vi "system.vi"() -> ()   [LabVIEW 2011]
uses:
  <vilib>/httpClient/POSTBuffer.vi
  <vilib>/httpClient/LabVIEWHTTPClient.lvlib
panel:
  in  "odswiez":bool
  in  "usunZdjecia":bool
  in  "usunZdjecie":bool
  in  "restartSystemu":bool
  in  "stopSystemu":bool
  in  "startSystemu":bool
  out "statusSystemu":bool
  in  "usunAlarmy":bool
  in  "usunAlarm":bool
  in  "alarmyRing":u16(ring) items=["2015-02-03 14:53:43"]
  out "picturesDir":string
  out "konfiguracja":string[][](array[string])
  out "alarmyString":string
  out "zdjecie":picture
  in  "zdjeciaRing":u16(ring) items=["2015-02-03 14:53:43.556413.jpg", "2015-02-03 14:53:45.230714.jpg", "2015-02-03 14:53:45.560907.jpg", "2015-02-03 14:53:45.893951.jpg", "2015-02-03 14:53:46.227903.jpg", "2015-02-03 14:53:46.565637.jpg", "2015-02-03 14:53:46.897487.jpg", "2015-02-03 14:53:47.231445.jpg", "2015-02-03 14:53:47.565422.jpg", "2015-02-03 14:53:47.899491.jpg", "2015-02-03 14:53:48.233446.jpg", "2015-02-03 14:53:48.567392.jpg", "2015-02-03 14:53:48.901593.jpg", "2015-02-03 14:53:49.235569.jpg", "2015-02-03 14:53:49.569530.jpg", "2015-02-03 14:53:49.903480.jpg", "2015-02-03 14:53:50.256797.jpg", "2015-02-03 14:53:50.571229.jpg", "2015-02-03 14:53:50.905749.jpg", "2015-02-03 14:53:51.239702.jpg", "2015-02-03 14:53:51.573789.jpg", "2015-02-03 14:53:51.907839.jpg"]
  in  "Zapisz":bool
  in  "edytujKonfiguracje":u16(ring) items=["logAlarms", "sendEmail", "senderEmail", "receiverEmail", "emailSubject", "picturesPerSecond"]
  in  "edytujKonfiguracje":string
  in  "Polacz":bool
  in  "Hasło:":string
  in  "Login:":string
  in  "IP:":string
  # "Przeglądaj zdjęcia:"
  # "Status systemu:"
  # "Wykryte alarmy:"
  # "Konfiguracja:"
  # "Zarządzaj alarmami:"
  # "Zarządzaj konfiguracją:"
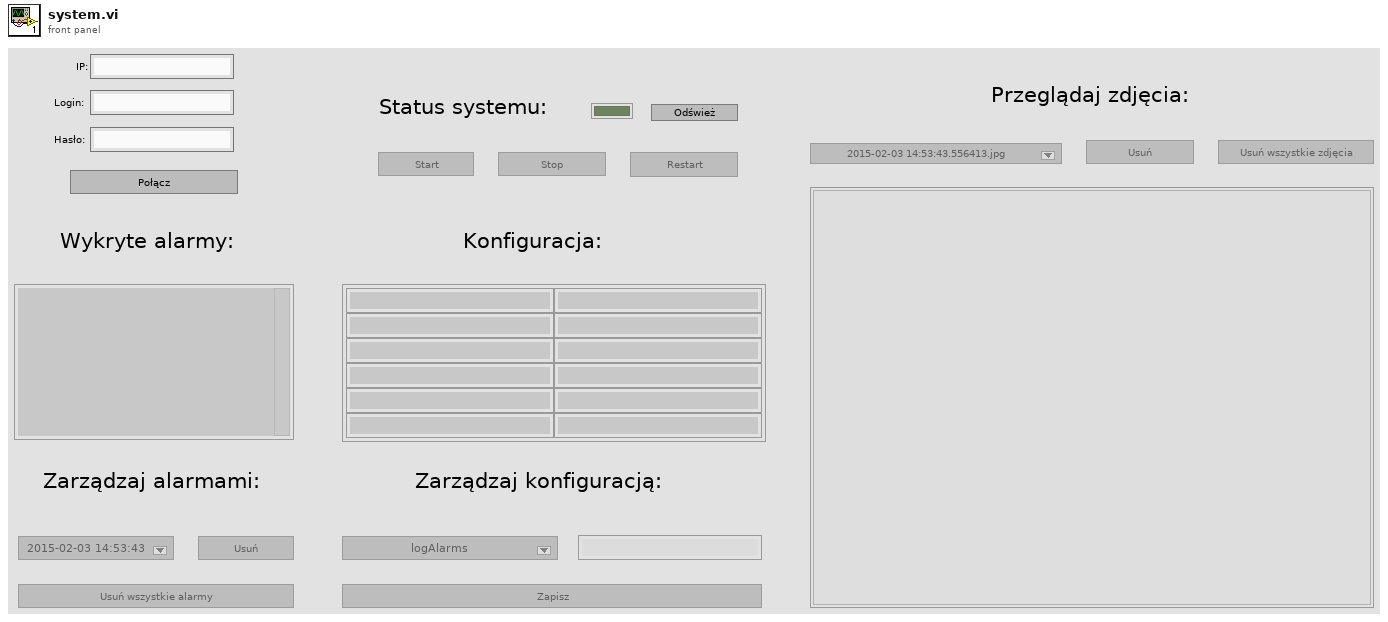
[diagram p1: front panel]
types:
  T1 = enum8{"Enabled", "Disabled", "Disabled and Grayed Out"}
  T2 = enum16{"open", "open or create", "create or replace", "create", "open (read only)"}
  T3 = typedef "LVBoundsTypeDef.ctl" = cluster{"Width":u32, "Height":u32}
  T4 = typedef "imagedata.ctl" = cluster{"image type":i32, "image depth":i32, "image":u8[], "mask":u8[], "colors":u32[], "Rectangle":cluster{"left":i16, "top":i16, "right":i16, "bottom":i16}}
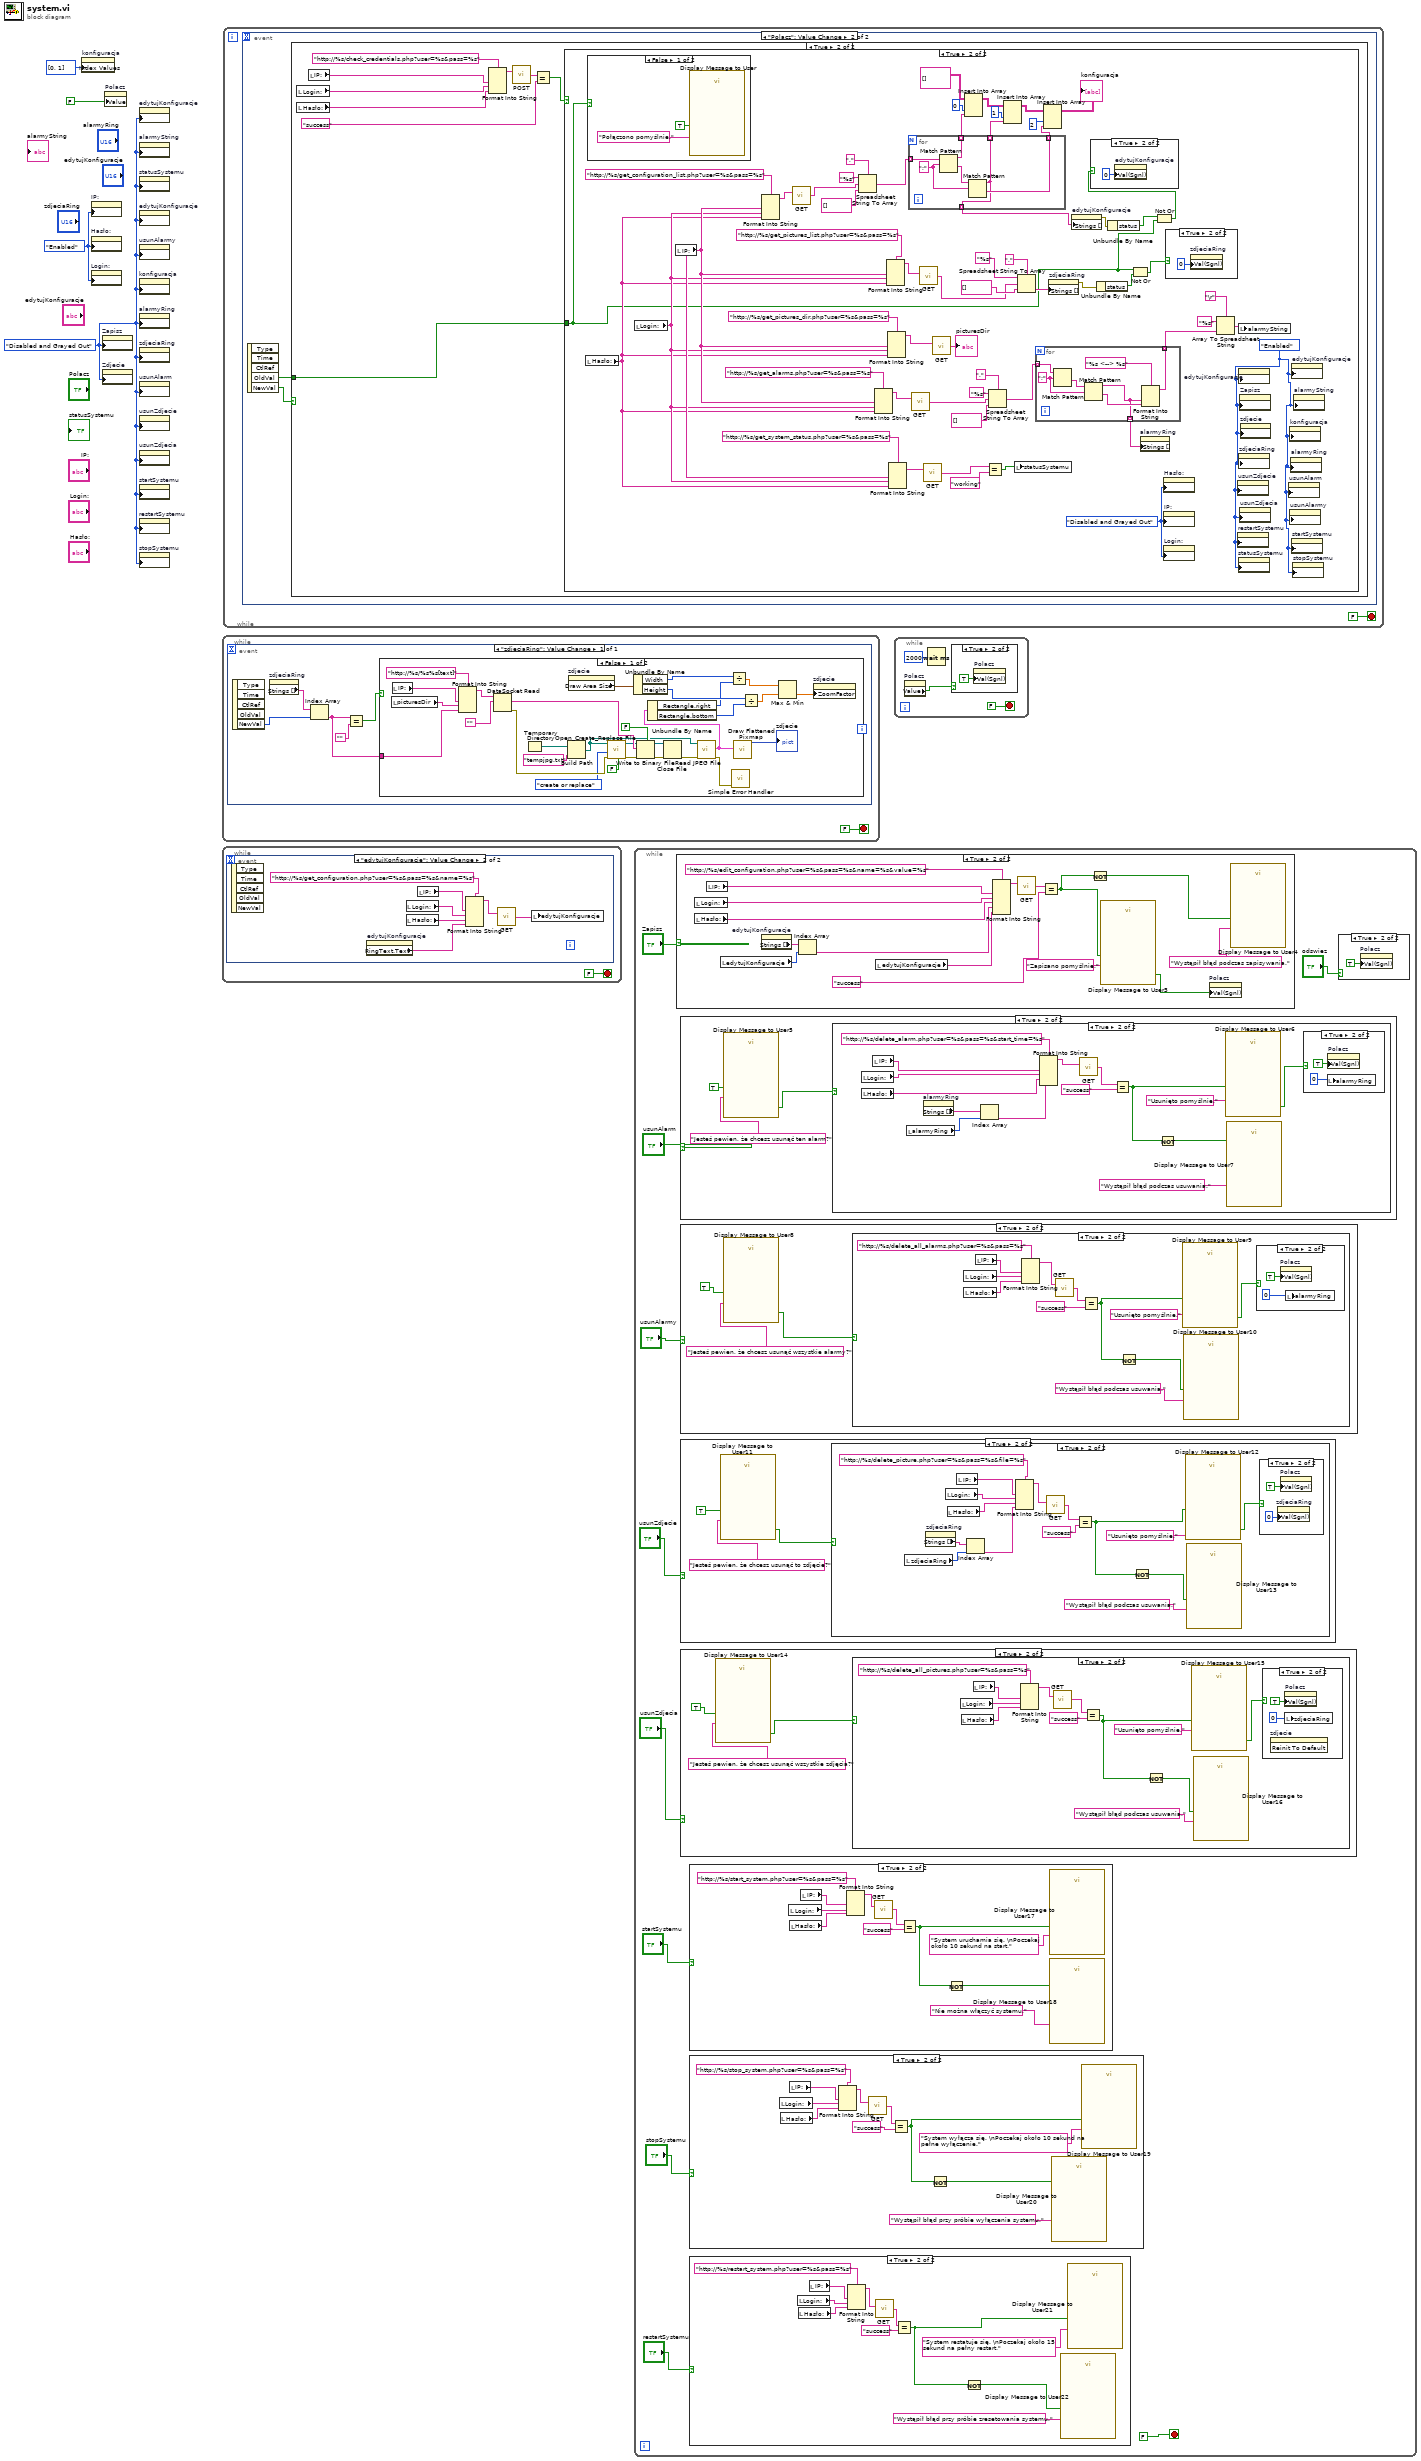
[diagram p0: block diagram]
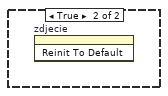
[diagram p3: hidden frame]
diagram:
  w2 = T1."Disabled and Grayed Out" ("Disabled")
  w4 = T1."Enabled" ("Disabled")
  n1 = property on="konfiguracja" class="Arr (strict)"("Index Values"=u32[] [0, 1]) -> ()  [unwired: 2 in, 2 out]
  n2 = property on="IP:" class="Str"("DisabledEnum"=w4) -> ()  [unwired: 2 in, 2 out]
  n3 = property on="Hasło:" class="Str"("DisabledEnum"=w4) -> ()  [unwired: 2 in, 2 out]
  n4 = property on="Login:" class="Str"("DisabledEnum"=w4) -> ()  [unwired: 2 in, 2 out]
  n5 = property on="Zapisz" class="Bool"("DisabledEnum"=w2) -> ()  [unwired: 2 in, 2 out]
  n6 = property on="Zdjecie" class="Pict"("DisabledEnum"=w2) -> ()  [unwired: 2 in, 2 out]
  n7 = property on="Polacz" class="Bool (strict)"("Value"=FALSE ("Polacz")) -> ()  [unwired: 2 in, 2 out]
  n8 = property on="edytujKonfiguracje" class="Str"("DisabledEnum"=w2) -> ()  [unwired: 2 in, 2 out]
  n9 = property on="alarmyString" class="Str"("DisabledEnum"=w2) -> ()  [unwired: 2 in, 2 out]
  n10 = property on="statusSystemu" class="Bool (strict)"("DisabledEnum"=w2) -> ()  [unwired: 2 in, 2 out]
  n11 = property on="edytujKonfiguracje" class="Ring (strict)"("DisabledEnum"=w2) -> ()  [unwired: 2 in, 2 out]
  n12 = property on="usunAlarmy" class="Bool"("DisabledEnum"=w2) -> ()  [unwired: 2 in, 2 out]
  n13 = property on="konfiguracja" class="Arr (strict)"("DisabledEnum"=w2) -> ()  [unwired: 2 in, 2 out]
  n14 = property on="alarmyRing" class="Ring (strict)"("DisabledEnum"=w2) -> ()  [unwired: 2 in, 2 out]
  n15 = property on="zdjeciaRing" class="Ring (strict)"("DisabledEnum"=w2) -> ()  [unwired: 2 in, 2 out]
  n16 = property on="usunAlarm" class="Bool"("DisabledEnum"=w2) -> ()  [unwired: 2 in, 2 out]
  n17 = property on="usunZdjecie" class="Bool"("DisabledEnum"=w2) -> ()  [unwired: 2 in, 2 out]
  n18 = property on="usunZdjecia" class="Bool"("DisabledEnum"=w2) -> ()  [unwired: 2 in, 2 out]
  n19 = property on="startSystemu" class="Bool"("DisabledEnum"=w2) -> ()  [unwired: 2 in, 2 out]
  n20 = property on="restartSystemu" class="Bool"("DisabledEnum"=w2) -> ()  [unwired: 2 in, 2 out]
  n21 = property on="stopSystemu" class="Bool"("DisabledEnum"=w2) -> ()  [unwired: 2 in, 2 out]
  n22 = while {
    stop <- FALSE stop-if-true
    n23 = event shown="[0] \"zdjeciaRing\": Value Change" {
      selector: _ -> [_]
      dyn-events: _ -> [_]
      timeout: _ -> [_]
      event "zdjeciaRing": Value Change {
        n24 = event-data() -> ("NewVal"=w9:u16)  [unwired: 1 in, 4 out]
        n25 = property on="zdjeciaRing" class="Ring (strict)"() -> ("Strings []"=w10:string[])  [unwired: 2 in, 2 out]
        n26 = Index Array(array=w10, index=w9) -> (element=w7:string)
        n27 = Equal?(x=w7, y="") -> (x = y?=w6:bool)
        n28 = case shown="False" w6 {
          tunnel: w7 -> [w11 _]
          frame False {
            n29 = local read "picturesDir"() -> (w14:string)
            n30 = local read "IP:"() -> (w15:string)
            n31 = Format Into String(format string="http://%s/%s%s[text]", w15, w14, w11) -> (resulting string=w12:string)  [unwired: 2 in, 1 out]
            n32 = DataSocket Read(10:"", 11:w12) -> (0:w37:errorcluster, 2:w28:string)  [unwired: 3 in, 5 out]
            n33 = Temporary Directory() -> (w25:path)
            n34 = Build Path(base path=w25, name or relative path="tempjpg.txt") -> (appended path=w36:path)
            n35 = property on="zdjecie" class="Pict"() -> ("Draw Area Size"=w23:T3)  [unwired: 2 in, 2 out]
            n36 = call <vilib>:"Open_Create_Replace File.vi"("advisory dialog? (display:T)"=FALSE, "error in (no error)"=w37, "function (open:0)"=T2."create or replace", "file path"=w36) -> ("error out"=w29:errorcluster, "refnum"=w27:refnum<file>)  [unwired: 3 in, 3 out]
            n37 = Unbundle By Name(w23) -> ("Width"=w22:u32, "Height"=w21:u32)
            n38 = Write to Binary File(file (use dialog)=w27, data=w28, error in=w29, 5:FALSE ("prepend array or string size? (T)")) -> (refnum out=w31:refnum<file>, error out=w32:errorcluster)  [unwired: 3 out]
            n39 = Close File(refnum=w31, error in=w32) -> (error out=w33:errorcluster)  [unwired: 1 out]
            n40 = call <vilib>:"Read JPEG File.vi"("error in (no error)"=w33, "path to JPEG file"=w36) -> ("error out"=w30:errorcluster, "image data"=w40:T4)  [unwired: 8 out]
            n41 = Unbundle By Name(w40) -> ("Rectangle.right"=w19:i16, "Rectangle.bottom"=w20:i16)
            n42 = Divide(x=w22, y=w19) -> (x/y=w18:dbl)
            n43 = call <vilib>:"Simple Error Handler.vi"("error in (no error)"=w30) -> ()  [unwired: 1 in, 8 out]
            n44 = call <vilib>:"Draw Flattened Pixmap.vi"("image data"=w40) -> ("new picture"=→"zdjecie":picture)  [unwired: 3 in, 5 out]
            n45 = Divide(x=w21, y=w20) -> (x/y=w17:dbl)
            n46 = Max & Min(x=w18, y=w17) -> (min(x,y)=w16:dbl)  [unwired: 1 out]
            n47 = property on="zdjecie" class="Pict"("ZoomFactor"=w16) -> ()  [unwired: 2 in, 2 out]
          }
          frame True {
            n48 = invoke on="zdjecie" class="Pict" method="Reinit To Default"() -> ()  [unwired: 3 in, 3 out]
          }
        }
      }
    }
  }
  n49 = while {
    stop <- FALSE stop-if-true
    n50 = event shown="[1] \"edytujKonfiguracje\": Value Change" {
      selector: _ -> [_ _]
      dyn-events: _ -> [_ _]
      timeout: _ -> [_ _]
      event Timeout {
        n51 = event-data() -> ()  [unwired: 1 in, 2 out]
      }
      event "edytujKonfiguracje": Value Change {
        n52 = event-data() -> ()  [unwired: 1 in, 5 out]
        n53 = property on="edytujKonfiguracje" class="Ring (strict)"() -> ("RingText.Text"=w47:string)  [unwired: 2 in, 2 out]
        n54 = local read "Login:"() -> (w45:string)
        n55 = local read "Hasło:"() -> (w44:string)
        n56 = local read "IP:"() -> (w46:string)
        n57 = Format Into String(format string="http://%s/get_configuration.php?user=%s&pass=%s&name=%s" ("http URL"), w46, w45, w44, w47) -> (resulting string=w43:string)  [unwired: 2 in, 1 out]
        n58 = call <vilib>:"GET.vi"("url"=w43) -> ("body"=w42:string)  [unwired: 11 in, 3 out]
        n59 = local write "edytujKonfiguracje"(w42) -> ()
      }
    }
  }
  n60 = while {
    stop <- FALSE stop-if-true
    n61 = event shown="[1] \"Polacz\": Value Change" {
      selector: _ -> [_ _]
      dyn-events: _ -> [_ _]
      timeout: _ -> [_ _]
      event Timeout {
        n62 = event-data() -> ()  [unwired: 1 in, 2 out]
      }
      event "Polacz": Value Change {
        n63 = event-data() -> ("OldVal"=w50:bool, "NewVal"=w51:bool)  [unwired: 1 in, 3 out]
        n64 = case shown="True" w51 {
          tunnel: w50 -> [_ w54]
          frame False {
            w52 = T1."Disabled and Grayed Out" ("Disabled")
            w53 = T1."Enabled" ("Disabled")
            n65 = property on="Hasło:" class="Str"("DisabledEnum"=w53) -> ()  [unwired: 2 in, 2 out]
            n66 = property on="Login:" class="Str"("DisabledEnum"=w53) -> ()  [unwired: 2 in, 2 out]
            n67 = property on="IP:" class="Str"("DisabledEnum"=w53) -> ()  [unwired: 2 in, 2 out]
            n68 = property on="stopSystemu" class="Bool"("DisabledEnum"=w52) -> ()  [unwired: 2 in, 2 out]
            n69 = property on="restartSystemu" class="Bool"("DisabledEnum"=w52) -> ()  [unwired: 2 in, 2 out]
            n70 = property on="statusSystemu" class="Bool (strict)"("DisabledEnum"=w52) -> ()  [unwired: 2 in, 2 out]
            n71 = property on="alarmyRing" class="Ring (strict)"("DisabledEnum"=w52) -> ()  [unwired: 2 in, 2 out]
            n72 = property on="startSystemu" class="Bool"("DisabledEnum"=w52) -> ()  [unwired: 2 in, 2 out]
            n73 = property on="zdjecie" class="Pict"("DisabledEnum"=w52) -> ()  [unwired: 2 in, 2 out]
            n74 = property on="konfiguracja" class="Arr (strict)"("DisabledEnum"=w52) -> ()  [unwired: 2 in, 2 out]
            n75 = property on="edytujKonfiguracje" class="Str"("DisabledEnum"=w52) -> ()  [unwired: 2 in, 2 out]
            n76 = property on="zdjeciaRing" class="Ring (strict)"("DisabledEnum"=w52) -> ()  [unwired: 2 in, 2 out]
            n77 = property on="edytujKonfiguracje" class="Ring (strict)"("DisabledEnum"=w52) -> ()  [unwired: 2 in, 2 out]
            n78 = property on="usunAlarm" class="Bool"("DisabledEnum"=w52) -> ()  [unwired: 2 in, 2 out]
            n79 = property on="alarmyString" class="Str"("DisabledEnum"=w52) -> ()  [unwired: 2 in, 2 out]
            n80 = property on="usunZdjecie" class="Bool"("DisabledEnum"=w52) -> ()  [unwired: 2 in, 2 out]
            n81 = property on="usunAlarmy" class="Bool"("DisabledEnum"=w52) -> ()  [unwired: 2 in, 2 out]
            n82 = property on="usunZdjecia" class="Bool"("DisabledEnum"=w52) -> ()  [unwired: 2 in, 2 out]
            n83 = property on="Zapisz" class="Bool"("DisabledEnum"=w52) -> ()  [unwired: 2 in, 2 out]
          }
          frame True {
            n84 = local read "Login:"() -> (w59:string)
            n85 = local read "Hasło:"() -> (w58:string)
            n86 = local read "IP:"() -> (w60:string)
            n87 = Format Into String(format string="http://%s/check_credentials.php?user=%s&pass=%s" ("url"), w60, w59, w58) -> (resulting string=w62:string)  [unwired: 2 in, 1 out]
            n88 = call-poly <vilib>:"POST.vi"("url"=w62) -> ("body"=w55:string)  [unwired: 11 in, 3 out]
            n89 = Equal?(x=w55, y="success") -> (x = y?=w56:bool)
            n90 = case shown="True" w56 {
              tunnel: w54 -> [_ w65]
              frame False {
                n91 = call "Display Message to User2"("Enable"=TRUE, "Message"="Wystąpił błąd podczas próby połączenia z systemem.") -> ()  [unwired: 8 in, 2 out]
              }
              frame True {
                w71 = T1."Disabled and Grayed Out" ("Disabled")
                w70 = T1."Enabled" ("Disabled")
                n92 = local read "Hasło:"() -> (w76:string)
                n93 = case shown="False" w65 {
                  frame False {
                    n94 = call "Display Message to User"("Enable"=TRUE, "Message"="Połączono pomyślnie.") -> ()  [unwired: 8 in, 2 out]
                  }
                  frame True {
                  }
                }
                n95 = local read "Login:"() -> (w77:string)
                n96 = local read "IP:"() -> (w78:string)
                n97 = Format Into String(format string="http://%s/get_configuration_list.php?user=%s&pass=%s" ("url"), w78, w77, w76) -> (resulting string=w97:string)  [unwired: 2 in, 1 out]
                n98 = call <vilib>:"GET.vi"("url"=w97) -> ("body"=w98:string)  [unwired: 11 in, 3 out]
                n99 = Spreadsheet String To Array(delimiter (Tab)=",", format string="%s", spreadsheet string=w98, array type (2D Dbl)=string[] []) -> (array=w116:string[])
                n100 = Format Into String(format string="http://%s/get_alarms.php?user=%s&pass=%s" ("url"), w78, w77, w76) -> (resulting string=w91:string)  [unwired: 2 in, 1 out]
                n101 = Format Into String(format string="http://%s/get_pictures_list.php?user=%s&pass=%s" ("http URL"), w78, w77, w76) -> (resulting string=w100:string)  [unwired: 2 in, 1 out]
                n102 = Format Into String(format string="http://%s/get_pictures_dir.php?user=%s&pass=%s" ("http URL"), w78, w77, w76) -> (resulting string=w95:string)  [unwired: 2 in, 1 out]
                n103 = Format Into String(format string="http://%s/get_system_status.php?user=%s&pass=%s" ("url"), w78, w77, w76) -> (resulting string=w75:string)  [unwired: 2 in, 1 out]
                n104 = for {
                  tunnel: w116 -> [w138] mode=indexing
                  tunnel: [w134] -> w115 mode=indexing
                  tunnel: [w133] -> w113 mode=indexing
                  tunnel: [w136] -> w111 mode=indexing
                  tunnel: [w133] -> w109 mode=indexing
                  w137 = ";" ("regular expression")
                  n105 = Match Pattern(string=w138, regular expression=w137) -> (before substring=w134:string, after substring=w135:string)  [unwired: 1 in, 2 out]
                  n106 = Match Pattern(string=w135, regular expression=w137) -> (before substring=w133:string, after substring=w136:string)  [unwired: 1 in, 2 out]
                }
                n107 = call <vilib>:"GET.vi"("url"=w91) -> ("body"=w86:string)  [unwired: 11 in, 3 out]
                n108 = call <vilib>:"GET.vi"("url"=w100) -> ("body"=w93:string)  [unwired: 11 in, 3 out]
                n109 = call <vilib>:"GET.vi"("url"=w75) -> ("body"=w74:string)  [unwired: 11 in, 3 out]
                n110 = call <vilib>:"GET.vi"("url"=w95) -> ("body"=→"picturesDir":string)  [unwired: 11 in, 3 out]
                n111 = Insert Into Array(array=string[][] [], index (col)=0 ("index (row)"), new element=w115) -> (w114:string[][])  [unwired: 1 in]
                n112 = Equal?(x=w74, y="working") -> (x = y?=w72:bool)
                n113 = Spreadsheet String To Array(delimiter (Tab)=",", format string="%s", spreadsheet string=w86, array type (2D Dbl)=string[] []) -> (array=w85:string[])
                n114 = Insert Into Array(array=w114, index (col)=1 ("index (row)"), new element=w113) -> (w112:string[][])  [unwired: 1 in]
                n115 = local write "statusSystemu"(w72) -> ()
                n116 = Spreadsheet String To Array(delimiter (Tab)=",", format string="%s" ("spreadsheet string"), spreadsheet string=w93, array type (2D Dbl)=string[] []) -> (array=w99:string[])
                n117 = for {
                  tunnel: w85 -> [w130] mode=indexing
                  tunnel: [w126] -> w84 mode=indexing
                  tunnel: [w124] -> w80 mode=indexing
                  w128 = ";" ("regular expression")
                  n118 = Match Pattern(string=w130, regular expression=w128) -> (after substring=w129:string)  [unwired: 1 in, 3 out]
                  n119 = Match Pattern(string=w129, regular expression=w128) -> (before substring=w124:string, after substring=w125:string)  [unwired: 1 in, 2 out]
                  n120 = Format Into String(format string="%s <--> %s", w124, w125) -> (resulting string=w126:string)  [unwired: 2 in, 1 out]
                }
                n121 = Insert Into Array(array=w112, index (col)=2 ("index (row)"), new element=w111) -> (→"konfiguracja":string[][])  [unwired: 1 in]
                n122 = property on="zdjeciaRing" class="Ring (strict)"("Strings []"=w99) -> (error out=w102:errorcluster)  [unwired: 2 in, 1 out]
                n123 = property on="edytujKonfiguracje" class="Ring (strict)"("Strings []"=w109) -> (error out=w90:errorcluster)  [unwired: 2 in, 1 out]
                n124 = Unbundle By Name(w102) -> ("status"=w67:bool)
                n125 = Unbundle By Name(w90) -> ("status"=w69:bool)
                n126 = Not Or(1:w67, 2:w65) -> (0:w66:bool)
                n127 = property on="alarmyRing" class="Ring (strict)"("Strings []"=w80) -> ()  [unwired: 2 in, 2 out]
                n128 = Not Or(1:w65, 2:w69) -> (0:w68:bool)
                n129 = case shown="True" w68 {
                  frame False {
                  }
                  frame True {
                    n130 = property on="edytujKonfiguracje" class="Ring (strict)"("Val(Sgnl)"=u16 0 ("Value (Signaling)")) -> ()  [unwired: 2 in, 2 out]
                  }
                }
                n131 = property on="Hasło:" class="Str"("DisabledEnum"=w71) -> ()  [unwired: 2 in, 2 out]
                n132 = property on="IP:" class="Str"("DisabledEnum"=w71) -> ()  [unwired: 2 in, 2 out]
                n133 = property on="Login:" class="Str"("DisabledEnum"=w71) -> ()  [unwired: 2 in, 2 out]
                n134 = case shown="True" w66 {
                  frame False {
                  }
                  frame True {
                    n135 = property on="zdjeciaRing" class="Ring (strict)"("Val(Sgnl)"=u16 0 ("Value (Signaling)")) -> ()  [unwired: 2 in, 2 out]
                  }
                }
                n136 = Array To Spreadsheet String(delimiter (Tab)="\r", array=w84, 3:"%s" ("format string")) -> (spreadsheet string=w81:string)
                n137 = property on="usunZdjecie" class="Bool"("DisabledEnum"=w70) -> ()  [unwired: 2 in, 2 out]
                n138 = property on="restartSystemu" class="Bool"("DisabledEnum"=w70) -> ()  [unwired: 2 in, 2 out]
                n139 = local write "alarmyString"(w81) -> ()
                n140 = property on="statusSystemu" class="Bool (strict)"("DisabledEnum"=w70) -> ()  [unwired: 2 in, 2 out]
                n141 = property on="edytujKonfiguracje" class="Ring (strict)"("DisabledEnum"=w70) -> ()  [unwired: 2 in, 2 out]
                n142 = property on="zdjeciaRing" class="Ring (strict)"("DisabledEnum"=w70) -> ()  [unwired: 2 in, 2 out]
                n143 = property on="Zapisz" class="Bool"("DisabledEnum"=w70) -> ()  [unwired: 2 in, 2 out]
                n144 = property on="usunZdjecia" class="Bool"("DisabledEnum"=w70) -> ()  [unwired: 2 in, 2 out]
                n145 = property on="zdjecie" class="Pict"("DisabledEnum"=w70) -> ()  [unwired: 2 in, 2 out]
                n146 = property on="usunAlarm" class="Bool"("DisabledEnum"=w70) -> ()  [unwired: 2 in, 2 out]
                n147 = property on="konfiguracja" class="Arr (strict)"("DisabledEnum"=w70) -> ()  [unwired: 2 in, 2 out]
                n148 = property on="usunAlarmy" class="Bool"("DisabledEnum"=w70) -> ()  [unwired: 2 in, 2 out]
                n149 = property on="alarmyRing" class="Ring (strict)"("DisabledEnum"=w70) -> ()  [unwired: 2 in, 2 out]
                n150 = property on="edytujKonfiguracje" class="Str"("DisabledEnum"=w70) -> ()  [unwired: 2 in, 2 out]
                n151 = property on="startSystemu" class="Bool"("DisabledEnum"=w70) -> ()  [unwired: 2 in, 2 out]
                n152 = property on="stopSystemu" class="Bool"("DisabledEnum"=w70) -> ()  [unwired: 2 in, 2 out]
                n153 = property on="alarmyString" class="Str"("DisabledEnum"=w70) -> ()  [unwired: 2 in, 2 out]
              }
            }
          }
        }
      }
    }
  }
  n154 = while {
    stop <- FALSE stop-if-true
    n155 = case shown="True" "Zapisz" {
      frame False {
      }
      frame True {
        n156 = local read "Login:"() -> (w268:string)
        n157 = local read "Hasło:"() -> (w267:string)
        n158 = local read "IP:"() -> (w269:string)
        n159 = local read "edytujKonfiguracje"() -> (w271:u16)
        n160 = property on="edytujKonfiguracje" class="Ring (strict)"() -> ("Strings []"=w270:string[])  [unwired: 2 in, 2 out]
        n161 = Index Array(array=w270, index=w271) -> (element=w258:string)
        n162 = local read "edytujKonfiguracje"() -> (w259:string)
        n163 = Format Into String(format string="http://%s/edit_configuration.php?user=%s&pass=%s&name=%s&value=%s" ("url"), w269, w268, w267, w258, w259) -> (resulting string=w265:string)  [unwired: 2 in, 1 out]
        n164 = call <vilib>:"GET.vi"("url"=w265) -> ("body"=w264:string)  [unwired: 11 in, 3 out]
        n165 = Equal?(x=w264, y="success") -> (x = y?=w261:bool)
        n166 = Not(x=w261) -> (.not. x?=w260:bool)
        n167 = call "Display Message to User3"("Enable"=w261, "Message"="Zapisano pomyślnie.") -> ("OK"=w257:bool)  [unwired: 8 in, 1 out]
        n168 = property on="Polacz" class="Bool (strict)"("Val(Sgnl)"=w257) -> ()  [unwired: 2 in, 2 out]
        n169 = call "Display Message to User4"("Enable"=w260, "Message"="Wystąpił błąd podczas zapisywania.") -> ()  [unwired: 8 in, 2 out]
      }
    }
    n170 = case shown="True" "usunAlarm" {
      frame False {
      }
      frame True {
        n171 = call "Display Message to User5"("Enable"=TRUE, "Message"="Jesteś pewien, że chcesz usunąć ten alarm?") -> ("Tak"=w237:bool)  [unwired: 8 in, 1 out]
        n172 = case shown="True" w237 {
          frame False {
          }
          frame True {
            n173 = local read "Login:"() -> (w252:string)
            n174 = local read "Hasło:"() -> (w251:string)
            n175 = local read "IP:"() -> (w253:string)
            n176 = local read "alarmyRing"() -> (w249:u16)
            n177 = property on="alarmyRing" class="Ring (strict)"() -> ("Strings []"=w250:string[])  [unwired: 2 in, 2 out]
            n178 = Index Array(array=w250, index=w249) -> (element=w248:string)
            n179 = Format Into String(format string="http://%s/delete_alarm.php?user=%s&pass=%s&start_time=%s" ("url"), w253, w252, w251, w248) -> (resulting string=w247:string)  [unwired: 2 in, 1 out]
            n180 = call <vilib>:"GET.vi"("url"=w247) -> ("body"=w246:string)  [unwired: 11 in, 3 out]
            n181 = Equal?(x=w246, y="success") -> (x = y?=w241:bool)
            n182 = Not(x=w241) -> (.not. x?=w242:bool)
            n183 = call "Display Message to User6"("Enable"=w241, "Message"="Usunięto pomyślnie.") -> ("OK"=w240:bool)  [unwired: 8 in, 1 out]
            n184 = call "Display Message to User7"("Enable"=w242, "Message"="Wystąpił błąd podczas usuwania.") -> ()  [unwired: 8 in, 2 out]
            n185 = case shown="True" w240 {
              frame False {
              }
              frame True {
                n186 = local write "alarmyRing"(0) -> ()
                n187 = property on="Polacz" class="Bool (strict)"("Val(Sgnl)"=TRUE ("Value (Signaling)")) -> ()  [unwired: 2 in, 2 out]
              }
            }
          }
        }
      }
    }
    n188 = case shown="True" "usunAlarmy" {
      frame False {
      }
      frame True {
        n189 = call "Display Message to User8"("Enable"=TRUE, "Message"="Jesteś pewien, że chcesz usunąć wszystkie alarmy?") -> ("Tak"=w220:bool)  [unwired: 8 in, 1 out]
        n190 = case shown="True" w220 {
          frame False {
          }
          frame True {
            n191 = local read "Login:"() -> (w232:string)
            n192 = local read "Hasło:"() -> (w231:string)
            n193 = local read "IP:"() -> (w233:string)
            n194 = Format Into String(format string="http://%s/delete_all_alarms.php?user=%s&pass=%s" ("url"), w233, w232, w231) -> (resulting string=w228:string)  [unwired: 2 in, 1 out]
            n195 = call <vilib>:"GET.vi"("url"=w228) -> ("body"=w230:string)  [unwired: 11 in, 3 out]
            n196 = Equal?(x=w230, y="success") -> (x = y?=w224:bool)
            n197 = Not(x=w224) -> (.not. x?=w225:bool)
            n198 = call "Display Message to User9"("Enable"=w224, "Message"="Usunięto pomyślnie.") -> ("OK"=w223:bool)  [unwired: 8 in, 1 out]
            n199 = call "Display Message to User10"("Enable"=w225, "Message"="Wystąpił błąd podczas usuwania.") -> ()  [unwired: 8 in, 2 out]
            n200 = case shown="True" w223 {
              frame False {
              }
              frame True {
                n201 = property on="Polacz" class="Bool (strict)"("Val(Sgnl)"=TRUE ("Value (Signaling)")) -> ()  [unwired: 2 in, 2 out]
                n202 = local write "alarmyRing"(0) -> ()
              }
            }
          }
        }
      }
    }
    n203 = case shown="True" "usunZdjecie" {
      frame False {
      }
      frame True {
        n204 = call "Display Message to User11"("Enable"=TRUE, "Message"="Jesteś pewien, że chcesz usunąć to zdjęcie?") -> ("Tak"=w200:bool)  [unwired: 8 in, 1 out]
        n205 = case shown="True" w200 {
          frame False {
          }
          frame True {
            n206 = local read "zdjeciaRing"() -> (w213:u16)
            n207 = property on="zdjeciaRing" class="Ring (strict)"() -> ("Strings []"=w212:string[])  [unwired: 2 in, 2 out]
            n208 = local read "Login:"() -> (w215:string)
            n209 = local read "Hasło:"() -> (w214:string)
            n210 = local read "IP:"() -> (w216:string)
            n211 = Index Array(array=w212, index=w213) -> (element=w211:string)
            n212 = Format Into String(format string="http://%s/delete_picture.php?user=%s&pass=%s&file=%s" ("url"), w216, w215, w214, w211) -> (resulting string=w210:string)  [unwired: 2 in, 1 out]
            n213 = call <vilib>:"GET.vi"("url"=w210) -> ("body"=w209:string)  [unwired: 11 in, 3 out]
            n214 = Equal?(x=w209, y="success") -> (x = y?=w204:bool)
            n215 = Not(x=w204) -> (.not. x?=w205:bool)
            n216 = call "Display Message to User12"("Enable"=w204, "Message"="Usunięto pomyślnie.") -> ("OK"=w203:bool)  [unwired: 8 in, 1 out]
            n217 = call "Display Message to User13"("Enable"=w205, "Message"="Wystąpił błąd podczas usuwania.") -> ()  [unwired: 8 in, 2 out]
            n218 = case shown="True" w203 {
              frame False {
              }
              frame True {
                n219 = property on="zdjeciaRing" class="Ring (strict)"("Val(Sgnl)"=u16 0 ("Value (Signaling)")) -> ()  [unwired: 2 in, 2 out]
                n220 = property on="Polacz" class="Bool (strict)"("Val(Sgnl)"=TRUE ("Value (Signaling)")) -> ()  [unwired: 2 in, 2 out]
              }
            }
          }
        }
      }
    }
    n221 = case shown="True" "usunZdjecia" {
      frame False {
      }
      frame True {
        n222 = call "Display Message to User14"("Enable"=TRUE, "Message"="Jesteś pewien, że chcesz usunąć wszystkie zdjęcia?") -> ("Tak"=w183:bool)  [unwired: 8 in, 1 out]
        n223 = case shown="True" w183 {
          frame False {
          }
          frame True {
            n224 = local read "Login:"() -> (w192:string)
            n225 = local read "Hasło:"() -> (w191:string)
            n226 = local read "IP:"() -> (w193:string)
            n227 = Format Into String(format string="http://%s/delete_all_pictures.php?user=%s&pass=%s" ("url"), w193, w192, w191) -> (resulting string=w195:string)  [unwired: 2 in, 1 out]
            n228 = call <vilib>:"GET.vi"("url"=w195) -> ("body"=w194:string)  [unwired: 11 in, 3 out]
            n229 = Equal?(x=w194, y="success") -> (x = y?=w187:bool)
            n230 = Not(x=w187) -> (.not. x?=w188:bool)
            n231 = call "Display Message to User15"("Enable"=w187, "Message"="Usunięto pomyślnie.") -> ("OK"=w186:bool)  [unwired: 8 in, 1 out]
            n232 = call "Display Message to User16"("Enable"=w188, "Message"="Wystąpił błąd podczas usuwania.") -> ()  [unwired: 8 in, 2 out]
            n233 = case shown="True" w186 {
              frame False {
              }
              frame True {
                n234 = invoke on="zdjecie" class="Pict" method="Reinit To Default"() -> ()  [unwired: 3 in, 3 out]
                n235 = property on="Polacz" class="Bool (strict)"("Val(Sgnl)"=TRUE ("Value (Signaling)")) -> ()  [unwired: 2 in, 2 out]
                n236 = local write "zdjeciaRing"(u16 0 ("Value (Signaling)")) -> ()
              }
            }
          }
        }
      }
    }
    n237 = case shown="True" "startSystemu" {
      frame False {
      }
      frame True {
        n238 = local read "Login:"() -> (w179:string)
        n239 = local read "Hasło:"() -> (w178:string)
        n240 = local read "IP:"() -> (w180:string)
        n241 = Format Into String(format string="http://%s/start_system.php?user=%s&pass=%s" ("url"), w180, w179, w178) -> (resulting string=w177:string)  [unwired: 2 in, 1 out]
        n242 = call <vilib>:"GET.vi"("url"=w177) -> ("body"=w175:string)  [unwired: 11 in, 3 out]
        n243 = Equal?(x=w175, y="success") -> (x = y?=w171:bool)
        n244 = Not(x=w171) -> (.not. x?=w172:bool)
        n245 = call "Display Message to User17"("Enable"=w171, "Message"="System uruchamia się. \nPoczekaj około 10 sekund na start.") -> ()  [unwired: 8 in, 2 out]
        n246 = call "Display Message to User18"("Enable"=w172, "Message"="Nie można włączyć systemu.") -> ()  [unwired: 8 in, 2 out]
      }
    }
    n247 = case shown="True" "stopSystemu" {
      frame False {
      }
      frame True {
        n248 = local read "Login:"() -> (w161:string)
        n249 = local read "Hasło:"() -> (w160:string)
        n250 = local read "IP:"() -> (w162:string)
        n251 = Format Into String(format string="http://%s/stop_system.php?user=%s&pass=%s" ("url"), w162, w161, w160) -> (resulting string=w167:string)  [unwired: 2 in, 1 out]
        n252 = call <vilib>:"GET.vi"("url"=w167) -> ("body"=w169:string)  [unwired: 11 in, 3 out]
        n253 = Equal?(x=w169, y="success") -> (x = y?=w163:bool)
        n254 = Not(x=w163) -> (.not. x?=w164:bool)
        n255 = call "Display Message to User20"("Enable"=w164, "Message"="Wystąpił błąd przy próbie wyłączenia systemu.") -> ()  [unwired: 8 in, 2 out]
        n256 = call "Display Message to User19"("Enable"=w163, "Message"="System wyłącza się. \nPoczekaj około 10 sekund na pełne wyłączenie.") -> ()  [unwired: 8 in, 2 out]
      }
    }
    n257 = case shown="True" "restartSystemu" {
      frame False {
      }
      frame True {
        n258 = local read "Login:"() -> (w157:string)
        n259 = local read "Hasło:"() -> (w156:string)
        n260 = local read "IP:"() -> (w158:string)
        n261 = Format Into String(format string="http://%s/restart_system.php?user=%s&pass=%s" ("url"), w158, w157, w156) -> (resulting string=w153:string)  [unwired: 2 in, 1 out]
        n262 = call <vilib>:"GET.vi"("url"=w153) -> ("body"=w154:string)  [unwired: 11 in, 3 out]
        n263 = Equal?(x=w154, y="success") -> (x = y?=w149:bool)
        n264 = Not(x=w149) -> (.not. x?=w150:bool)
        n265 = call "Display Message to User22"("Enable"=w150, "Message"="Wystąpił błąd przy próbie zresetowania systemu.") -> ()  [unwired: 8 in, 2 out]
        n266 = call "Display Message to User21"("Enable"=w149, "Message"="System restatuje się. \nPoczekaj około 15 sekund na pełny restart.") -> ()  [unwired: 8 in, 2 out]
      }
    }
    n267 = case shown="True" "odswiez" {
      frame False {
      }
      frame True {
        n268 = property on="Polacz" class="Bool (strict)"("Val(Sgnl)"=TRUE ("Value (Signaling)")) -> ()  [unwired: 2 in, 2 out]
      }
    }
  }
  n269 = while {
    stop <- FALSE stop-if-true
    n270 = property on="Polacz" class="Bool (strict)"() -> ("Value"=w273:bool)  [unwired: 2 in, 2 out]
    n271 = Wait (ms)(milliseconds to wait=u32 2000) -> ()  [unwired: 1 out]
    n272 = case shown="True" w273 {
      frame False {
      }
      frame True {
        n273 = property on="Polacz" class="Bool (strict)"("Val(Sgnl)"=TRUE ("Value (Signaling)")) -> ()  [unwired: 2 in, 2 out]
      }
    }
  }
